vi "Main.vi"(7 "sweep rate, /min":dbl=0.2, 8 "sweep to:":dbl=4.0, 9 "sweep":T8(radio)=enum."2636a_smub") -> ()   [LabVIEW 2021] (continued)
                    n293 = property on="iTC_addr_hyper" class="VISAName"() -> ("Value"=w276:refnum<visa-resource-name>)  [unwired: 2 in, 2 out]
                    n294 = call "iTCread.vi"("VISA resource name"=w276, "iTCreadCtrl"=iTCreadCtrl."Sample Temp") -> ("number"=w277:dbl)  [unwired: 5 in, 3 out]
                  }
                }
                n295 = property on="Hyper Channel" class="DigNum (strict)"("Value"=w243) -> ()  [unwired: 2 in, 2 out]
              }
            }
          }
          frame #3 {
            # "Update current value of measured channel"
            n296 = property on="Monitor" class="Bool (strict)"() -> ("Value"=w279:bool)  [unwired: 2 in, 2 out]
            n297 = case shown="True" w279 {
              frame False {
              }
              frame True {
                n298 = stacked-sequence {
                  frame #0 {
                    # "Prepare the display format"
                    n299 = local read "2636A smua meas v"() -> (w285:bool)
                    n300 = local read "2636A smub meas v"() -> (w283:bool)
                    n301 = local read "2636A smub meas i"() -> (w282:bool)
                    n302 = local read "2636A smua meas i"() -> (w284:bool)
                    n303 = property on="sweep" class="RadioBtnsControl (strict)"() -> ("Value"=w280:T8)  [unwired: 2 in, 2 out]
                    n304 = Compound Arithmetic op=OR(w285, w284, w283, w282) -> (w281:bool)
                    n305 = case shown="True" w281 {
                      frame False {
                      }
                      frame True {
                        # "opens session for 2636a system sourcemeter"
                        n306 = local read "2614A addr"() -> (w340:refnum<visa-resource-name>)
                        n307 = VISA Close(VISA resource name=w340) -> ()  [unwired: 1 in, 1 out]
                      }
                    }
                    n308 = case shown="\"AuxOut0\"" w280 {
                      frame "2400_1" {
                        # "add label for the first column in the datafile"
                        n309 = stacked-sequence {
                          frame #0 {
                            n310 = property on="data_caption" class="Str"("Value"="") -> ()  [unwired: 2 in, 2 out]
                            n311 = property on="Figure_axis" class="Arr (strict)"("Value"=string[] [] ("Figure_axis_string")) -> ()  [unwired: 2 in, 2 out]
                          }
                          frame #1 {
                            w288 = "V_sweep_2400_1" ("V_sweep")
                            n312 = Concatenate Strings(w288, "\t") -> (w290:string)
                            n313 = Build Array(w288) -> (w289:string[])
                            n314 = property on="data_caption" class="Str"("Value"=w290) -> ()  [unwired: 2 in, 2 out]
                            n315 = property on="Figure_axis" class="Arr (strict)"("Value"=w289) -> ()  [unwired: 2 in, 2 out]
                          }
                        }
                      }
                      frame "2400_2" {
                        n316 = stacked-sequence {
                          frame #0 {
                            n317 = property on="data_caption" class="Str"("Value"="") -> ()  [unwired: 2 in, 2 out]
                            n318 = property on="Figure_axis" class="Arr (strict)"("Value"=string[] [] ("Figure_axis_string")) -> ()  [unwired: 2 in, 2 out]
                          }
                          frame #1 {
                            w294 = "V_sweep_2400_2" ("V_sweep")
                            n319 = Build Array(w294) -> (w295:string[])
                            n320 = Concatenate Strings(w294, "\t") -> (w297:string)
                            n321 = property on="Figure_axis" class="Arr (strict)"("Value"=w295) -> ()  [unwired: 2 in, 2 out]
                            n322 = property on="data_caption" class="Str"("Value"=w297) -> ()  [unwired: 2 in, 2 out]
                          }
                        }
                      }
                      frame "2400_3" {
                        n323 = stacked-sequence {
                          frame #0 {
                            n324 = property on="data_caption" class="Str"("Value"="") -> ()  [unwired: 2 in, 2 out]
                            n325 = property on="Figure_axis" class="Arr (strict)"("Value"=string[] [] ("Figure_axis_string")) -> ()  [unwired: 2 in, 2 out]
                          }
                          frame #1 {
                            w300 = "V_sweep_2400_3" ("V_sweep")
                            n326 = Concatenate Strings(w300, "\t") -> (w303:string)
                            n327 = Build Array(w300) -> (w301:string[])
                            n328 = property on="data_caption" class="Str"("Value"=w303) -> ()  [unwired: 2 in, 2 out]
                            n329 = property on="Figure_axis" class="Arr (strict)"("Value"=w301) -> ()  [unwired: 2 in, 2 out]
                          }
                        }
                      }
                      frame "2636a_smua" {
                        n330 = stacked-sequence {
                          frame #0 {
                            n331 = property on="data_caption" class="Str"("Value"="") -> ()  [unwired: 2 in, 2 out]
                            n332 = property on="Figure_axis" class="Arr (strict)"("Value"=string[] [] ("Figure_axis_string")) -> ()  [unwired: 2 in, 2 out]
                          }
                          frame #1 {
                            w306 = "V_sweep_2636a_smua" ("V_sweep")
                            n333 = Concatenate Strings(w306, "\t") -> (w309:string)
                            n334 = Build Array(w306) -> (w307:string[])
                            n335 = property on="data_caption" class="Str"("Value"=w309) -> ()  [unwired: 2 in, 2 out]
                            n336 = property on="Figure_axis" class="Arr (strict)"("Value"=w307) -> ()  [unwired: 2 in, 2 out]
                          }
                        }
                      }
                      frame "2636a_smub" {
                        n337 = stacked-sequence {
                          frame #0 {
                            n338 = property on="data_caption" class="Str"("Value"="") -> ()  [unwired: 2 in, 2 out]
                            n339 = property on="Figure_axis" class="Arr (strict)"("Value"=string[] [] ("Figure_axis_string")) -> ()  [unwired: 2 in, 2 out]
                          }
                          frame #1 {
                            w312 = "V_sweep_2636a_smub" ("V_sweep")
                            n340 = Build Array(w312) -> (w313:string[])
                            n341 = Concatenate Strings(w312, "\t") -> (w315:string)
                            n342 = property on="Figure_axis" class="Arr (strict)"("Value"=w313) -> ()  [unwired: 2 in, 2 out]
                            n343 = property on="data_caption" class="Str"("Value"=w315) -> ()  [unwired: 2 in, 2 out]
                          }
                        }
                      }
                      frame "time_sweep", Default {
                        n344 = stacked-sequence {
                          frame #0 {
                            n345 = property on="data_caption" class="Str"("Value"="") -> ()  [unwired: 2 in, 2 out]
                            n346 = property on="Figure_axis" class="Arr (strict)"("Value"=string[] [] ("Figure_axis_string")) -> ()  [unwired: 2 in, 2 out]
                          }
                          frame #1 {
                            w318 = "time_sweep" ("V_sweep")
                            n347 = Build Array(w318) -> (w319:string[])
                            n348 = Concatenate Strings(w318, "\t") -> (w320:string)
                            n349 = property on="Figure_axis" class="Arr (strict)"("Value"=w319) -> ()  [unwired: 2 in, 2 out]
                            n350 = property on="data_caption" class="Str"("Value"=w320) -> ()  [unwired: 2 in, 2 out]
                          }
                        }
                      }
                      frame "iPS" {
                        # "sweep iPS"
                        n351 = stacked-sequence {
                          frame #0 {
                            n352 = property on="data_caption" class="Str"("Value"="") -> ()  [unwired: 2 in, 2 out]
                            n353 = property on="Figure_axis" class="Arr (strict)"("Value"=string[] [] ("Figure_axis_string")) -> ()  [unwired: 2 in, 2 out]
                          }
                          frame #1 {
                            w324 = "iPS_OutputField" ("V_sweep")
                            n354 = Build Array(w324) -> (w325:string[])
                            n355 = Concatenate Strings(w324, "\t") -> (w327:string)
                            n356 = property on="Figure_axis" class="Arr (strict)"("Value"=w325) -> ()  [unwired: 2 in, 2 out]
                            n357 = property on="data_caption" class="Str"("Value"=w327) -> ()  [unwired: 2 in, 2 out]
                          }
                        }
                      }
                      frame "iTC" {
                        n358 = stacked-sequence {
                          frame #0 {
                            n359 = property on="data_caption" class="Str"("Value"="") -> ()  [unwired: 2 in, 2 out]
                            n360 = property on="Figure_axis" class="Arr (strict)"("Value"=string[] ["", "SR830_1_ip", "SR830_1_oop", "SR830_2_ip", "SR830_2_oop", "2461_meas_v", "2461_meas_i", "2636A_smua_v", "2636A_smua_i", "formula"] ("Figure_axis")) -> ()  [unwired: 2 in, 2 out]
                          }
                          frame #1 {
                            w332 = "iTC_sample"
                            n361 = Build Array(w332) -> (w331:string[])
                            n362 = Concatenate Strings(w332, "\t") -> (w330:string)
                            n363 = property on="data_caption" class="Str"("Value"=w330) -> ()  [unwired: 2 in, 2 out]
                            n364 = property on="Figure_axis" class="Arr (strict)"("Value"=w331) -> ()  [unwired: 2 in, 2 out]
                          }
                        }
                      }
                      frame "AuxOut0" {
                        n365 = stacked-sequence {
                          frame #0 {
                            n366 = property on="data_caption" class="Str"("Value"="") -> ()  [unwired: 2 in, 2 out]
                            n367 = property on="Figure_axis" class="Arr (strict)"("Value"=string[] ["", "SR830_1_ip", "SR830_1_oop", "SR830_2_ip", "SR830_2_oop", "2461_meas_v", "2461_meas_i", "2636A_smua_v", "2636A_smua_i", "formula"] ("Figure_axis")) -> ()  [unwired: 2 in, 2 out]
                          }
                          frame #1 {
                            w338 = "V_sweep_AuxOut0"
                            n368 = Build Array(w338) -> (w337:string[])
                            n369 = Concatenate Strings(w338, "\t") -> (w336:string)
                            n370 = property on="data_caption" class="Str"("Value"=w336) -> ()  [unwired: 2 in, 2 out]
                            n371 = property on="Figure_axis" class="Arr (strict)"("Value"=w337) -> ()  [unwired: 2 in, 2 out]
                          }
                        }
                      }
                    }
                  }
                  frame #1 {
                    # "0 = SR830_1_ip\n1 = SR830_1_oop\n2 = SR830_2_ip\n3 = SR830_2_oop\n4 = SR830_3_ip\n5 = SR830_3_oop\n6 = SR830_4_ip \n7 = SR830_4_oop \n8= 2400_1_v \n9 = 2400_1_i \n10 = 2400_2_v\n11 = 2400_2_i \n12 = 2400_3_v \n13 = 2400_3_i \n14 = 2182A_1_ch1 \n15 = 2182A_1_ch2 \n16 = 2182A_2_ch1 \n17 = 2182A_2_ch2\n18 = 2182A_3_ch1 \n19 = 2182A_3_ch2 \n20 = 2182A_4_ch1 \n21 = 2182A_4_ch2 \n22 = 2636A_smua_v \n23 = 2636A_smua_i \n24 = 2636A_smub_v \n25 = 2636A_smub_i \n26 = time\n27 = iPS_Field\n28 = iPS_Magnet_T\n29 = iPS__SH_T\n30 = iTC _sample_T\n31 = iTC _VTI_T\n32 = iTC _PT1_T\n33 = iTC _PT2_T\n34 = iTC _VTI_P"
                    # "this part constructs the first (text) line for the data file with names of all measured variables,\nalso constructs a text array contaning names of all measured variable for the \"ring\" (so parameter can be selected and plotted)"
                    n372 = stacked-sequence {
                      frame #0 {
                        # "SR830 1 in phase (SR830_1_ip)"
                        n373 = local read "SR830 1 ip"() -> (w345:bool)
                        n374 = property on="Figure_axis" class="Arr (strict)"() -> ("Value"=w342:string[])  [unwired: 2 in, 2 out]
                        n375 = property on="data_caption" class="Str"() -> ("Value"=w344:string)  [unwired: 2 in, 2 out]
                        n376 = case shown="True" w345 {
                          tunnel: w344 -> [w347 w353]
                          tunnel: [w347 w352] -> w343
                          tunnel: w342 -> [w346 w350]
                          tunnel: [w346 w348] -> w341
                          frame False {
                            # "not measure SR830 1 in phase signal (SR830_1_ip)"
                          }
                          frame True {
                            w349 = "SR830_1_ip"
                            # "measure SR830 1 in phase signal (SR830_1_ip)"
                            n377 = local read "SR830 1 addr"() -> (w354:u8)
                            n378 = Number To Decimal String(number=w354) -> (decimal integer string=w355:string)  [unwired: 1 in]
                            n379 = GPIB Clear(3:w355) -> ()  [unwired: 1 in, 2 out]
                            n380 = Build Array (concatenate)(w350, w349) -> (w348:string[])
                            n381 = Concatenate Strings(w353, w349, "\t") -> (w352:string)
                          }
                        }
                        n382 = property on="Figure_axis" class="Arr (strict)"("Value"=w341) -> ()  [unwired: 2 in, 2 out]
                        n383 = property on="data_caption" class="Str"("Value"=w343) -> ()  [unwired: 2 in, 2 out]
                      }
                      frame #1 {
                        # "SR830 1 out of phase (SR830_1_oop)"
                        n384 = local read "SR830 1 oop"() -> (w360:bool)
                        n385 = property on="Figure_axis" class="Arr (strict)"() -> ("Value"=w357:string[])  [unwired: 2 in, 2 out]
                        n386 = property on="data_caption" class="Str"() -> ("Value"=w359:string)  [unwired: 2 in, 2 out]
                        n387 = case shown="False" w360 {
                          tunnel: w359 -> [w362 w368]
                          tunnel: [w362 w367] -> w358
                          tunnel: w357 -> [w361 w365]
                          tunnel: [w361 w363] -> w356
                          frame False {
                            # "not measure SR830 1 out of phase signal (SR830_1_oop)"
                          }
                          frame True {
                            w364 = "SR830_1_oop"
                            # "measure SR830 1 out of phase signal (SR830_1_oop)"
                            n388 = local read "SR830 1 addr"() -> (w369:u8)
                            n389 = Number To Decimal String(number=w369) -> (decimal integer string=w370:string)  [unwired: 1 in]
                            n390 = GPIB Clear(3:w370) -> ()  [unwired: 1 in, 2 out]
                            n391 = Build Array (concatenate)(w365, w364) -> (w363:string[])
                            n392 = Concatenate Strings(w368, w364, "\t") -> (w367:string)
                          }
                        }
                        n393 = property on="Figure_axis" class="Arr (strict)"("Value"=w356) -> ()  [unwired: 2 in, 2 out]
                        n394 = property on="data_caption" class="Str"("Value"=w358) -> ()  [unwired: 2 in, 2 out]
                      }
                      frame #2 {
                        # "SR830 2 in phase (SR830_2_ip)"
                        n395 = local read "SR830 2 ip"() -> (w375:bool)
                        n396 = property on="Figure_axis" class="Arr (strict)"() -> ("Value"=w372:string[])  [unwired: 2 in, 2 out]
                        n397 = property on="data_caption" class="Str"() -> ("Value"=w374:string)  [unwired: 2 in, 2 out]
                        n398 = case shown="True" w375 {
                          tunnel: w374 -> [w377 w383]
                          tunnel: [w377 w382] -> w373
                          tunnel: w372 -> [w376 w380]
                          tunnel: [w376 w378] -> w371
                          frame False {
                            # "not measure SR830 2 in phase signal (SR830_2_ip)"
                          }
                          frame True {
                            w379 = "SR830_2_ip"
                            # "measure SR830 2 in phase signal (SR830_2_ip)"
                            n399 = local read "SR830 2 addr"() -> (w384:u8)
                            n400 = Number To Decimal String(number=w384) -> (decimal integer string=w385:string)  [unwired: 1 in]
                            n401 = GPIB Clear(3:w385) -> ()  [unwired: 1 in, 2 out]
                            n402 = Build Array (concatenate)(w380, w379) -> (w378:string[])
                            n403 = Concatenate Strings(w383, w379, "\t") -> (w382:string)
                          }
                        }
                        n404 = property on="Figure_axis" class="Arr (strict)"("Value"=w371) -> ()  [unwired: 2 in, 2 out]
                        n405 = property on="data_caption" class="Str"("Value"=w373) -> ()  [unwired: 2 in, 2 out]
                      }
                      frame #3 {
                        # "SR830 2 out of phase (SR830_2_oop)"
                        n406 = local read "SR830 2 oop"() -> (w390:bool)
                        n407 = property on="Figure_axis" class="Arr (strict)"() -> ("Value"=w387:string[])  [unwired: 2 in, 2 out]
                        n408 = property on="data_caption" class="Str"() -> ("Value"=w389:string)  [unwired: 2 in, 2 out]
                        n409 = case shown="True" w390 {
                          tunnel: w389 -> [w392 w398]
                          tunnel: [w392 w397] -> w388
                          tunnel: w387 -> [w391 w395]
                          tunnel: [w391 w393] -> w386
                          frame False {
                            # "not measure SR830 2 out of phase signal (SR830_2_oop)"
                          }
                          frame True {
                            w394 = "SR830_2_oop"
                            # "measure SR830 2 out of phase signal (SR830_2_oop)"
                            n410 = local read "SR830 2 addr"() -> (w399:u8)
                            n411 = Number To Decimal String(number=w399) -> (decimal integer string=w400:string)  [unwired: 1 in]
                            n412 = GPIB Clear(3:w400) -> ()  [unwired: 1 in, 2 out]
                            n413 = Build Array (concatenate)(w395, w394) -> (w393:string[])
                            n414 = Concatenate Strings(w398, w394, "\t") -> (w397:string)
                          }
                        }
                        n415 = property on="Figure_axis" class="Arr (strict)"("Value"=w386) -> ()  [unwired: 2 in, 2 out]
                        n416 = property on="data_caption" class="Str"("Value"=w388) -> ()  [unwired: 2 in, 2 out]
                      }
                      frame #4 {
                        # "SR830 3 in phase (SR830_3_ip)"
                        n417 = local read "SR830 3 ip"() -> (w405:bool)
                        n418 = property on="Figure_axis" class="Arr (strict)"() -> ("Value"=w402:string[])  [unwired: 2 in, 2 out]
                        n419 = property on="data_caption" class="Str"() -> ("Value"=w404:string)  [unwired: 2 in, 2 out]
                        n420 = case shown="True" w405 {
                          tunnel: w404 -> [w407 w413]
                          tunnel: [w407 w412] -> w403
                          tunnel: w402 -> [w406 w410]
                          tunnel: [w406 w408] -> w401
                          frame False {
                            # "not measure SR830 3 in phase signal (SR830_3_ip)"
                          }
                          frame True {
                            w409 = "SR830_3_ip"
                            # "measure SR830 3 in phase signal (SR830_3_ip)"
                            n421 = local read "SR830 3 addr"() -> (w414:u8)
                            n422 = Number To Decimal String(number=w414) -> (decimal integer string=w415:string)  [unwired: 1 in]
                            n423 = GPIB Clear(3:w415) -> ()  [unwired: 1 in, 2 out]
                            n424 = Build Array (concatenate)(w410, w409) -> (w408:string[])
                            n425 = Concatenate Strings(w413, w409, "\t") -> (w412:string)
                          }
                        }
                        n426 = property on="Figure_axis" class="Arr (strict)"("Value"=w401) -> ()  [unwired: 2 in, 2 out]
                        n427 = property on="data_caption" class="Str"("Value"=w403) -> ()  [unwired: 2 in, 2 out]
                      }
                      frame #5 {
                        # "SR830 3 out of phase (SR830_3_oop)"
                        n428 = local read "SR830 3 oop"() -> (w420:bool)
                        n429 = property on="Figure_axis" class="Arr (strict)"() -> ("Value"=w417:string[])  [unwired: 2 in, 2 out]
                        n430 = property on="data_caption" class="Str"() -> ("Value"=w419:string)  [unwired: 2 in, 2 out]
                        n431 = case shown="True" w420 {
                          tunnel: w419 -> [w422 w428]
                          tunnel: [w422 w427] -> w418
                          tunnel: w417 -> [w421 w425]
                          tunnel: [w421 w423] -> w416
                          frame False {
                            # "not measure SR830 3 out of phase signal (SR830_3_oop)"
                          }
                          frame True {
                            w424 = "SR830_3_oop"
                            # "measure SR830 3 out phase signal (SR830_3_oop)"
                            n432 = local read "SR830 3 addr"() -> (w429:u8)
                            n433 = Number To Decimal String(number=w429) -> (decimal integer string=w430:string)  [unwired: 1 in]
                            n434 = GPIB Clear(3:w430) -> ()  [unwired: 1 in, 2 out]
                            n435 = Build Array (concatenate)(w425, w424) -> (w423:string[])
                            n436 = Concatenate Strings(w428, w424, "\t") -> (w427:string)
                          }
                        }
                        n437 = property on="Figure_axis" class="Arr (strict)"("Value"=w416) -> ()  [unwired: 2 in, 2 out]
                        n438 = property on="data_caption" class="Str"("Value"=w418) -> ()  [unwired: 2 in, 2 out]
                      }
                      frame #6 {
                        # "SR830 4 in phase (SR830_4_ip)"
                        n439 = local read "SR830 4 ip"() -> (w435:bool)
                        n440 = property on="Figure_axis" class="Arr (strict)"() -> ("Value"=w432:string[])  [unwired: 2 in, 2 out]
                        n441 = property on="data_caption" class="Str"() -> ("Value"=w434:string)  [unwired: 2 in, 2 out]
                        n442 = case shown="True" w435 {
                          tunnel: w434 -> [w437 w443]
                          tunnel: [w437 w442] -> w433
                          tunnel: w432 -> [w436 w440]
                          tunnel: [w436 w438] -> w431
                          frame False {
                            # "not measure SR830 4 in phase signal (SR830_4_ip)"
                          }
                          frame True {
                            w439 = "SR830_4_ip"
                            # "measure SR830 4 in phase signal (SR830_4_ip)"
                            n443 = local read "SR830 4 addr"() -> (w444:u8)
                            n444 = Number To Decimal String(number=w444) -> (decimal integer string=w445:string)  [unwired: 1 in]
                            n445 = GPIB Clear(3:w445) -> ()  [unwired: 1 in, 2 out]
                            n446 = Build Array (concatenate)(w440, w439) -> (w438:string[])
                            n447 = Concatenate Strings(w443, w439, "\t") -> (w442:string)
                          }
                        }
                        n448 = property on="Figure_axis" class="Arr (strict)"("Value"=w431) -> ()  [unwired: 2 in, 2 out]
                        n449 = property on="data_caption" class="Str"("Value"=w433) -> ()  [unwired: 2 in, 2 out]
                      }
                      frame #7 {
                        # "SR830 4 out of phase (SR830_4_oop)"
                        n450 = local read "SR830 4 oop"() -> (w450:bool)
                        n451 = property on="Figure_axis" class="Arr (strict)"() -> ("Value"=w447:string[])  [unwired: 2 in, 2 out]
                        n452 = property on="data_caption" class="Str"() -> ("Value"=w449:string)  [unwired: 2 in, 2 out]
                        n453 = case shown="True" w450 {
                          tunnel: w449 -> [w452 w458]
                          tunnel: [w452 w457] -> w448
                          tunnel: w447 -> [w451 w455]
                          tunnel: [w451 w453] -> w446
                          frame False {
                            # "not measure SR830 4 out of phase signal (SR830_4_oop)"
                          }
                          frame True {
                            w454 = "SR830_4_oop"
                            # "measure SR830 4 out of phase signal (SR830_4_oop)"
                            n454 = local read "SR830 4 addr"() -> (w459:u8)
                            n455 = Number To Decimal String(number=w459) -> (decimal integer string=w460:string)  [unwired: 1 in]
                            n456 = GPIB Clear(3:w460) -> ()  [unwired: 1 in, 2 out]
                            n457 = Build Array (concatenate)(w455, w454) -> (w453:string[])
                            n458 = Concatenate Strings(w458, w454, "\t") -> (w457:string)
                          }
                        }
                        n459 = property on="Figure_axis" class="Arr (strict)"("Value"=w446) -> ()  [unwired: 2 in, 2 out]
                        n460 = property on="data_caption" class="Str"("Value"=w448) -> ()  [unwired: 2 in, 2 out]
                      }
                      frame #8 {
                        # "2400 1 voltage measure (2400_1_v)"
                        n461 = local read "2400 1 meas v"() -> (w465:bool)
                        n462 = property on="Figure_axis" class="Arr (strict)"() -> ("Value"=w462:string[])  [unwired: 2 in, 2 out]
                        n463 = property on="data_caption" class="Str"() -> ("Value"=w464:string)  [unwired: 2 in, 2 out]
                        n464 = case shown="True" w465 {
                          tunnel: w464 -> [w467 w473]
                          tunnel: [w467 w472] -> w463
                          tunnel: w462 -> [w466 w470]
                          tunnel: [w466 w468] -> w461
                          frame False {
                            # "not measure 2400 1 voltage (2400_1_v)"
                          }
                          frame True {
                            w469 = "2400_1_v"
                            # "measure 2400 1 voltage (2400_1_v)"
                            n465 = local read "2400 1 addr"() -> (w474:u8)
                            n466 = Number To Decimal String(number=w474) -> (decimal integer string=w475:string)  [unwired: 1 in]
                            n467 = GPIB Clear(3:w475) -> ()  [unwired: 1 in, 2 out]
                            n468 = Build Array (concatenate)(w470, w469) -> (w468:string[])
                            n469 = Concatenate Strings(w473, w469, "\t") -> (w472:string)
                          }
                        }
                        n470 = property on="Figure_axis" class="Arr (strict)"("Value"=w461) -> ()  [unwired: 2 in, 2 out]
                        n471 = property on="data_caption" class="Str"("Value"=w463) -> ()  [unwired: 2 in, 2 out]
                      }
                      frame #9 {
                        # "2400 1 current measure (2400_1_i)"
                        n472 = local read "2400 1 meas i"() -> (w480:bool)
                        n473 = property on="Figure_axis" class="Arr (strict)"() -> ("Value"=w477:string[])  [unwired: 2 in, 2 out]
                        n474 = property on="data_caption" class="Str"() -> ("Value"=w479:string)  [unwired: 2 in, 2 out]
                        n475 = case shown="True" w480 {
                          tunnel: w479 -> [w482 w488]
                          tunnel: [w482 w487] -> w478
                          tunnel: w477 -> [w481 w485]
                          tunnel: [w481 w483] -> w476
                          frame False {
                            # "not measure 2400 1 current (2400_1_i)"
                          }
                          frame True {
                            w484 = "2400_1_i"
                            # "measure 2400 1 current (2400_1_i)"
                            n476 = local read "2400 1 addr"() -> (w489:u8)
                            n477 = Number To Decimal String(number=w489) -> (decimal integer string=w490:string)  [unwired: 1 in]
                            n478 = GPIB Clear(3:w490) -> ()  [unwired: 1 in, 2 out]
                            n479 = Build Array (concatenate)(w485, w484) -> (w483:string[])
                            n480 = Concatenate Strings(w488, w484, "\t") -> (w487:string)
                          }
                        }
                        n481 = property on="Figure_axis" class="Arr (strict)"("Value"=w476) -> ()  [unwired: 2 in, 2 out]
                        n482 = property on="data_caption" class="Str"("Value"=w478) -> ()  [unwired: 2 in, 2 out]
                      }
                      frame #10 {
                        # "2400 2 voltage measure (2400_2_v)"
                        n483 = local read "2400 2 meas v"() -> (w495:bool)
                        n484 = property on="Figure_axis" class="Arr (strict)"() -> ("Value"=w492:string[])  [unwired: 2 in, 2 out]
                        n485 = property on="data_caption" class="Str"() -> ("Value"=w494:string)  [unwired: 2 in, 2 out]
                        n486 = case shown="True" w495 {
                          tunnel: w494 -> [w497 w503]
                          tunnel: [w497 w502] -> w493
                          tunnel: w492 -> [w496 w500]
                          tunnel: [w496 w498] -> w491
                          frame False {
                            # "not measure 2400 2 voltage (2400_2_v)"
                          }
                          frame True {
                            w499 = "2400_2_v"
                            # "measure 2400 2 voltage (2400_2_v)"
                            n487 = local read "2400 2 addr"() -> (w504:u8)
                            n488 = Number To Decimal String(number=w504) -> (decimal integer string=w505:string)  [unwired: 1 in]
                            n489 = GPIB Clear(3:w505) -> ()  [unwired: 1 in, 2 out]
                            n490 = Build Array (concatenate)(w500, w499) -> (w498:string[])
                            n491 = Concatenate Strings(w503, w499, "\t") -> (w502:string)
                          }
                        }
                        n492 = property on="Figure_axis" class="Arr (strict)"("Value"=w491) -> ()  [unwired: 2 in, 2 out]
                        n493 = property on="data_caption" class="Str"("Value"=w493) -> ()  [unwired: 2 in, 2 out]
                      }
                      frame #11 {
                        # "2400 2 current measure (2400_2_i)"
                        n494 = local read "2400 2 meas i"() -> (w510:bool)
                        n495 = property on="Figure_axis" class="Arr (strict)"() -> ("Value"=w507:string[])  [unwired: 2 in, 2 out]
                        n496 = property on="data_caption" class="Str"() -> ("Value"=w509:string)  [unwired: 2 in, 2 out]
                        n497 = case shown="True" w510 {
                          tunnel: w509 -> [w512 w518]
                          tunnel: [w512 w517] -> w508
                          tunnel: w507 -> [w511 w515]
                          tunnel: [w511 w513] -> w506
                          frame False {
                            # "not measure 2400 2 current (2400_2_i)"
                          }
                          frame True {
                            w514 = "2400_2_i"
                            # "measure 2400 2 current (2400_2_i)"
                            n498 = local read "2400 2 addr"() -> (w519:u8)
                            n499 = Number To Decimal String(number=w519) -> (decimal integer string=w520:string)  [unwired: 1 in]
                            n500 = GPIB Clear(3:w520) -> ()  [unwired: 1 in, 2 out]
                            n501 = Build Array (concatenate)(w515, w514) -> (w513:string[])
                            n502 = Concatenate Strings(w518, w514, "\t") -> (w517:string)
                          }
                        }
                        n503 = property on="Figure_axis" class="Arr (strict)"("Value"=w506) -> ()  [unwired: 2 in, 2 out]
                        n504 = property on="data_caption" class="Str"("Value"=w508) -> ()  [unwired: 2 in, 2 out]
                      }
                      frame #12 {
                        # "2400 3 voltage measure (2400_3_v)"
                        n505 = local read "2400 3 meas v"() -> (w525:bool)
                        n506 = property on="Figure_axis" class="Arr (strict)"() -> ("Value"=w522:string[])  [unwired: 2 in, 2 out]
                        n507 = property on="data_caption" class="Str"() -> ("Value"=w524:string)  [unwired: 2 in, 2 out]
                        n508 = case shown="True" w525 {
                          tunnel: w524 -> [w527 w533]
                          tunnel: [w527 w532] -> w523
                          tunnel: w522 -> [w526 w530]
                          tunnel: [w526 w528] -> w521
                          frame False {
                            # "not measure 2400 3 voltage (2400_3_v)"
                          }
                          frame True {
                            w529 = "2400_3_v"
                            # "measure 2400 3 voltage (2400_3_v)"
                            n509 = local read "2400 3 addr"() -> (w534:u8)
                            n510 = Number To Decimal String(number=w534) -> (decimal integer string=w535:string)  [unwired: 1 in]
                            n511 = GPIB Clear(3:w535) -> ()  [unwired: 1 in, 2 out]
                            n512 = Build Array (concatenate)(w530, w529) -> (w528:string[])
                            n513 = Concatenate Strings(w533, w529, "\t") -> (w532:string)
                          }
                        }
                        n514 = property on="Figure_axis" class="Arr (strict)"("Value"=w521) -> ()  [unwired: 2 in, 2 out]
                        n515 = property on="data_caption" class="Str"("Value"=w523) -> ()  [unwired: 2 in, 2 out]
                      }
                      frame #13 {
                        # "2400 3 current measure (2400_3_i)"
                        n516 = local read "2400 3 meas i"() -> (w540:bool)
                        n517 = property on="Figure_axis" class="Arr (strict)"() -> ("Value"=w537:string[])  [unwired: 2 in, 2 out]
                        n518 = property on="data_caption" class="Str"() -> ("Value"=w539:string)  [unwired: 2 in, 2 out]
                        n519 = case shown="True" w540 {
                          tunnel: w539 -> [w542 w548]
                          tunnel: [w542 w547] -> w538
                          tunnel: w537 -> [w541 w545]
                          tunnel: [w541 w543] -> w536
                          frame False {
                            # "not measure 2400 3 current (2400_3_i)"
                          }
                          frame True {
                            w544 = "2400_3_i"
                            # "measure 2400 3 current (2400_3_i)"
                            n520 = local read "2400 3 addr"() -> (w549:u8)
                            n521 = Number To Decimal String(number=w549) -> (decimal integer string=w550:string)  [unwired: 1 in]
                            n522 = GPIB Clear(3:w550) -> ()  [unwired: 1 in, 2 out]
                            n523 = Build Array (concatenate)(w545, w544) -> (w543:string[])
                            n524 = Concatenate Strings(w548, w544, "\t") -> (w547:string)
                          }
                        }
                        n525 = property on="Figure_axis" class="Arr (strict)"("Value"=w536) -> ()  [unwired: 2 in, 2 out]
                        n526 = property on="data_caption" class="Str"("Value"=w538) -> ()  [unwired: 2 in, 2 out]
                      }
                      frame #14 {
                        # "2182A 1 channel 1 measure (2182A_1_ch1)"
                        n527 = local read "2182A 1 ch1"() -> (w555:bool)
                        n528 = property on="Figure_axis" class="Arr (strict)"() -> ("Value"=w552:string[])  [unwired: 2 in, 2 out]
                        n529 = property on="data_caption" class="Str"() -> ("Value"=w554:string)  [unwired: 2 in, 2 out]
                        n530 = case shown="False" w555 {
                          tunnel: w554 -> [w557 w563]
                          tunnel: [w557 w562] -> w553
                          tunnel: w552 -> [w556 w560]
                          tunnel: [w556 w558] -> w551
                          frame False {
                            # "not measure 2182A 1 channel 1 (2182A_1_ch1)"
                          }
                          frame True {
                            w559 = "2182A_1_ch1"
                            # "measure 2182A 1 channel 1 (2182A_1_ch1)"
                            n531 = local read "2182A 1 addr"() -> (w564:u8)
                            n532 = Number To Decimal String(number=w564) -> (decimal integer string=w565:string)  [unwired: 1 in]
                            n533 = GPIB Clear(3:w565) -> ()  [unwired: 1 in, 2 out]
                            n534 = Build Array (concatenate)(w560, w559) -> (w558:string[])
                            n535 = Concatenate Strings(w563, w559, "\t") -> (w562:string)
                          }
                        }
                        n536 = property on="Figure_axis" class="Arr (strict)"("Value"=w551) -> ()  [unwired: 2 in, 2 out]
                        n537 = property on="data_caption" class="Str"("Value"=w553) -> ()  [unwired: 2 in, 2 out]
                      }
                      frame #15 {
                        # "2182A 1 channel 2 measure (2182A_1_ch2)"
                        n538 = local read "2182A 1 ch2"() -> (w570:bool)
                        n539 = property on="Figure_axis" class="Arr (strict)"() -> ("Value"=w567:string[])  [unwired: 2 in, 2 out]
                        n540 = property on="data_caption" class="Str"() -> ("Value"=w569:string)  [unwired: 2 in, 2 out]
                        n541 = case shown="True" w570 {
                          tunnel: w569 -> [w572 w578]
                          tunnel: [w572 w577] -> w568
                          tunnel: w567 -> [w571 w575]
                          tunnel: [w571 w573] -> w566
                          frame False {
                            # "not measure 2182A 1 channel 2 (2182A_1_ch2)"
                          }
                          frame True {
                            w574 = "2182A_1_ch2"
                            # "measure 2182A 1 channel 2 (2182A_1_ch2)"
                            n542 = local read "2182A 1 addr"() -> (w579:u8)
                            n543 = Number To Decimal String(number=w579) -> (decimal integer string=w580:string)  [unwired: 1 in]
                            n544 = GPIB Clear(3:w580) -> ()  [unwired: 1 in, 2 out]
                            n545 = Build Array (concatenate)(w575, w574) -> (w573:string[])
                            n546 = Concatenate Strings(w578, w574, "\t") -> (w577:string)
                          }
                        }
                        n547 = property on="Figure_axis" class="Arr (strict)"("Value"=w566) -> ()  [unwired: 2 in, 2 out]
                        n548 = property on="data_caption" class="Str"("Value"=w568) -> ()  [unwired: 2 in, 2 out]
                      }
                      frame #16 {
                        # "2182A 2 channel 1 measure (2182A_2_ch1)"
                        n549 = local read "2182A 2 ch1"() -> (w585:bool)
                        n550 = property on="Figure_axis" class="Arr (strict)"() -> ("Value"=w582:string[])  [unwired: 2 in, 2 out]
                        n551 = property on="data_caption" class="Str"() -> ("Value"=w584:string)  [unwired: 2 in, 2 out]
                        n552 = case shown="True" w585 {
                          tunnel: w584 -> [w587 w593]
                          tunnel: [w587 w592] -> w583
                          tunnel: w582 -> [w586 w590]
                          tunnel: [w586 w588] -> w581
                          frame False {
                            # "not measure 2182A 2 channel 1 (2182A_2_ch1)"
                          }
                          frame True {
                            w589 = "2182A_2_ch1"
                            # "measure 2182A 2 channel 1 (2182A_2_ch1)"
                            n553 = local read "2182A 2 addr"() -> (w594:u8)
                            n554 = Number To Decimal String(number=w594) -> (decimal integer string=w595:string)  [unwired: 1 in]
                            n555 = GPIB Clear(3:w595) -> ()  [unwired: 1 in, 2 out]
                            n556 = Build Array (concatenate)(w590, w589) -> (w588:string[])
                            n557 = Concatenate Strings(w593, w589, "\t") -> (w592:string)
                          }
                        }
                        n558 = property on="Figure_axis" class="Arr (strict)"("Value"=w581) -> ()  [unwired: 2 in, 2 out]
                        n559 = property on="data_caption" class="Str"("Value"=w583) -> ()  [unwired: 2 in, 2 out]
                      }
                      frame #17 {
                        # "2182A 2 channel 2 measure (2182A_2_ch2)"
                        n560 = local read "2182A 2 ch2"() -> (w600:bool)
                        n561 = property on="Figure_axis" class="Arr (strict)"() -> ("Value"=w597:string[])  [unwired: 2 in, 2 out]
                        n562 = property on="data_caption" class="Str"() -> ("Value"=w599:string)  [unwired: 2 in, 2 out]
                        n563 = case shown="True" w600 {
                          tunnel: w599 -> [w602 w608]
                          tunnel: [w602 w607] -> w598
                          tunnel: w597 -> [w601 w605]
                          tunnel: [w601 w603] -> w596
                          frame False {
                            # "not measure 2182A 2 channel 2 (2182A_2_ch2)"
                          }
                          frame True {
                            w604 = "2182A_2_ch2"
                            # "measure 2182A 2 channel 2 (2182A_2_ch2)"
                            n564 = local read "2182A 2 addr"() -> (w609:u8)
                            n565 = Number To Decimal String(number=w609) -> (decimal integer string=w610:string)  [unwired: 1 in]
                            n566 = GPIB Clear(3:w610) -> ()  [unwired: 1 in, 2 out]
                            n567 = Build Array (concatenate)(w605, w604) -> (w603:string[])
                            n568 = Concatenate Strings(w608, w604, "\t") -> (w607:string)
                          }
                        }
                        n569 = property on="Figure_axis" class="Arr (strict)"("Value"=w596) -> ()  [unwired: 2 in, 2 out]
                        n570 = property on="data_caption" class="Str"("Value"=w598) -> ()  [unwired: 2 in, 2 out]
                      }
                      frame #18 {
                        # "2182A 3 channel 1 measure (2182A_3_ch1)"
                        n571 = local read "2182A 3 ch1"() -> (w615:bool)
                        n572 = property on="Figure_axis" class="Arr (strict)"() -> ("Value"=w612:string[])  [unwired: 2 in, 2 out]
                        n573 = property on="data_caption" class="Str"() -> ("Value"=w614:string)  [unwired: 2 in, 2 out]
                        n574 = case shown="True" w615 {
                          tunnel: w614 -> [w617 w623]
                          tunnel: [w617 w622] -> w613
                          tunnel: w612 -> [w616 w620]
                          tunnel: [w616 w618] -> w611
                          frame False {
                            # "not measure 2182A 3 channel 1 (2182A_3_ch1)"
                          }
                          frame True {
                            w619 = "2182A_3_ch1"
                            # "measure 2182A 3 channel 1 (2182A_3_ch1)"
                            n575 = local read "2182A 3 addr"() -> (w624:u8)
                            n576 = Number To Decimal String(number=w624) -> (decimal integer string=w625:string)  [unwired: 1 in]
                            n577 = GPIB Clear(3:w625) -> ()  [unwired: 1 in, 2 out]
                            n578 = Build Array (concatenate)(w620, w619) -> (w618:string[])
                            n579 = Concatenate Strings(w623, w619, "\t") -> (w622:string)
                          }
                        }
                        n580 = property on="Figure_axis" class="Arr (strict)"("Value"=w611) -> ()  [unwired: 2 in, 2 out]
                        n581 = property on="data_caption" class="Str"("Value"=w613) -> ()  [unwired: 2 in, 2 out]
                      }
                      frame #19 {
                        # "2182A 3 channel 2 measure (2182A_3_ch2)"
                        n582 = local read "2182A 3 ch2"() -> (w630:bool)
                        n583 = property on="Figure_axis" class="Arr (strict)"() -> ("Value"=w627:string[])  [unwired: 2 in, 2 out]
                        n584 = property on="data_caption" class="Str"() -> ("Value"=w629:string)  [unwired: 2 in, 2 out]
                        n585 = case shown="False" w630 {
                          tunnel: w629 -> [w632 w638]
                          tunnel: [w632 w637] -> w628
                          tunnel: w627 -> [w631 w635]
                          tunnel: [w631 w633] -> w626
                          frame False {
                            # "not measure 2182A 3 channel 2 (2182A_3_ch2)"
                          }
                          frame True {
                            w634 = "2182A_3_ch2"
                            # "measure 2182A 3 channel 2 (2182A_3_ch2)"
                            n586 = local read "2182A 3 addr"() -> (w639:u8)
                            n587 = Number To Decimal String(number=w639) -> (decimal integer string=w640:string)  [unwired: 1 in]
                            n588 = GPIB Clear(3:w640) -> ()  [unwired: 1 in, 2 out]
                            n589 = Build Array (concatenate)(w635, w634) -> (w633:string[])
                            n590 = Concatenate Strings(w638, w634, "\t") -> (w637:string)
                          }
                        }
                        n591 = property on="Figure_axis" class="Arr (strict)"("Value"=w626) -> ()  [unwired: 2 in, 2 out]
                        n592 = property on="data_caption" class="Str"("Value"=w628) -> ()  [unwired: 2 in, 2 out]
                      }
                      frame #20 {
                        # "2182A 4 channel 1 measure (2182A_4_ch1)"
                        n593 = local read "2182A 4 ch1"() -> (w645:bool)
                        n594 = property on="Figure_axis" class="Arr (strict)"() -> ("Value"=w642:string[])  [unwired: 2 in, 2 out]
                        n595 = property on="data_caption" class="Str"() -> ("Value"=w644:string)  [unwired: 2 in, 2 out]
                        n596 = case shown="True" w645 {
                          tunnel: w644 -> [w647 w653]
                          tunnel: [w647 w652] -> w643
                          tunnel: w642 -> [w646 w650]
                          tunnel: [w646 w648] -> w641
                          frame False {
                            # "not measure 2182A 4 channel 1 (2182A_4_ch1)"
                          }
                          frame True {
                            w649 = "2182A_4_ch1"
                            # "measure 2182A 4 channel 1 (2182A_4_ch1)"
                            n597 = local read "2182A 4 addr"() -> (w654:u8)
                            n598 = Number To Decimal String(number=w654) -> (decimal integer string=w655:string)  [unwired: 1 in]
                            n599 = GPIB Clear(3:w655) -> ()  [unwired: 1 in, 2 out]
                            n600 = Build Array (concatenate)(w650, w649) -> (w648:string[])
                            n601 = Concatenate Strings(w653, w649, "\t") -> (w652:string)
                          }
                        }
                        n602 = property on="Figure_axis" class="Arr (strict)"("Value"=w641) -> ()  [unwired: 2 in, 2 out]
                        n603 = property on="data_caption" class="Str"("Value"=w643) -> ()  [unwired: 2 in, 2 out]
                      }
                      frame #21 {
                        # "2182A 4 channel 2 measure (2182A_4_ch2)"
                        n604 = local read "2182A 4 ch2"() -> (w660:bool)
                        n605 = property on="Figure_axis" class="Arr (strict)"() -> ("Value"=w657:string[])  [unwired: 2 in, 2 out]
                        n606 = property on="data_caption" class="Str"() -> ("Value"=w659:string)  [unwired: 2 in, 2 out]
                        n607 = case shown="True" w660 {
                          tunnel: w659 -> [w662 w668]
                          tunnel: [w662 w667] -> w658
                          tunnel: w657 -> [w661 w665]
                          tunnel: [w661 w663] -> w656
                          frame False {
                            # "not measure 2182A 4 channel 2 (2182A_4_ch2)"
                          }
                          frame True {
                            w664 = "2182A_4_ch2"
                            # "measure 2182A 4 channel 2 (2182A_4_ch2)"
                            n608 = local read "2182A 4 addr"() -> (w669:u8)
                            n609 = Number To Decimal String(number=w669) -> (decimal integer string=w670:string)  [unwired: 1 in]
                            n610 = GPIB Clear(3:w670) -> ()  [unwired: 1 in, 2 out]
                            n611 = Build Array (concatenate)(w665, w664) -> (w663:string[])
                            n612 = Concatenate Strings(w668, w664, "\t") -> (w667:string)
                          }
                        }
                        n613 = property on="Figure_axis" class="Arr (strict)"("Value"=w656) -> ()  [unwired: 2 in, 2 out]
                        n614 = property on="data_caption" class="Str"("Value"=w658) -> ()  [unwired: 2 in, 2 out]
                      }
                      frame #22 {
                        # "2636A smua measure voltage (2636A_smua_v)"
                        n615 = local read "2636A smua meas v"() -> (w675:bool)
                        n616 = property on="Figure_axis" class="Arr (strict)"() -> ("Value"=w672:string[])  [unwired: 2 in, 2 out]
                        n617 = property on="data_caption" class="Str"() -> ("Value"=w674:string)  [unwired: 2 in, 2 out]
                        n618 = case shown="True" w675 {
                          tunnel: w674 -> [w677 w688]
                          tunnel: [w677 w687] -> w673
                          tunnel: w672 -> [w676 w685]
                          tunnel: [w676 w683] -> w671
                          frame False {
                            # "not measure voltage on 2636A smua (2636A_smua_v)"
                          }
                          frame True {
                            w684 = "2636A_smua_v"
                            # "measure voltage on 2636A smua (2636A_smua_v)"
                            n619 = local read "2614A addr"() -> (w679:refnum<visa-resource-name>)
                            n620 = VISA Open(VISA resource name=w679) -> (VISA resource name=w678:refnum<visa-resource-name>, error out=w680:errorcluster)  [unwired: 4 in]
                            n621 = VISA Clear(VISA resource name=w678, error in (no error)=w680) -> (VISA resource name out=w682:refnum<visa-resource-name>)  [unwired: 1 out]
                            n622 = property class="Instr"(reference=w682, "General Settings:Timeout Value"=u32 10000) -> ()  [unwired: 1 in, 2 out]
                            n623 = Build Array (concatenate)(w685, w684) -> (w683:string[])
                            n624 = Concatenate Strings(w688, w684, "\t") -> (w687:string)
                          }
                        }
                        n625 = property on="Figure_axis" class="Arr (strict)"("Value"=w671) -> ()  [unwired: 2 in, 2 out]
                        n626 = property on="data_caption" class="Str"("Value"=w673) -> ()  [unwired: 2 in, 2 out]
                      }
                      frame #23 {
                        # "2636A smua measure current (2636A_smua_i)"
                        n627 = local read "2636A smua meas i"() -> (w693:bool)
                        n628 = property on="Figure_axis" class="Arr (strict)"() -> ("Value"=w690:string[])  [unwired: 2 in, 2 out]
                        n629 = property on="data_caption" class="Str"() -> ("Value"=w692:string)  [unwired: 2 in, 2 out]
                        n630 = case shown="True" w693 {
                          tunnel: w692 -> [w695 w706]
                          tunnel: [w695 w705] -> w691
                          tunnel: w690 -> [w694 w703]
                          tunnel: [w694 w701] -> w689
                          frame False {
                            # "not measure current on 2636A smua (2636A_smua_i)"
                          }
                          frame True {
                            w702 = "2636A_smua_i"
                            # "measure current on 2636A smua (2636A_smua_i)"
                            n631 = local read "2614A addr"() -> (w698:refnum<visa-resource-name>)
                            n632 = VISA Open(VISA resource name=w698) -> (VISA resource name=w697:refnum<visa-resource-name>, error out=w696:errorcluster)  [unwired: 4 in]
                            n633 = VISA Clear(VISA resource name=w697, error in (no error)=w696) -> (VISA resource name out=w699:refnum<visa-resource-name>)  [unwired: 1 out]
                            n634 = Build Array (concatenate)(w703, w702) -> (w701:string[])
                            n635 = property class="Instr"(reference=w699, "General Settings:Timeout Value"=u32 10000) -> ()  [unwired: 1 in, 2 out]
                            n636 = Concatenate Strings(w706, w702, "\t") -> (w705:string)
                          }
                        }
                        n637 = property on="Figure_axis" class="Arr (strict)"("Value"=w689) -> ()  [unwired: 2 in, 2 out]
                        n638 = property on="data_caption" class="Str"("Value"=w691) -> ()  [unwired: 2 in, 2 out]
                      }
                      frame #24 {
                        # "2636A smub measure voltage (2636A_smub_v)"
                        n639 = local read "2636A smub meas v"() -> (w711:bool)
                        n640 = property on="Figure_axis" class="Arr (strict)"() -> ("Value"=w708:string[])  [unwired: 2 in, 2 out]
                        n641 = property on="data_caption" class="Str"() -> ("Value"=w710:string)  [unwired: 2 in, 2 out]
                        n642 = case shown="True" w711 {
                          tunnel: w710 -> [w713 w724]
                          tunnel: [w713 w723] -> w709
                          tunnel: w708 -> [w712 w721]
                          tunnel: [w712 w719] -> w707
                          frame False {
                            # "not measure voltage on 2636A smub (2636A_smub_v)"
                          }
                          frame True {
                            w720 = "2636A_smub_v"
                            # "measure voltage on 2636A smub (2636A_smub_v)"
                            n643 = local read "2614A addr"() -> (w715:refnum<visa-resource-name>)
                            n644 = VISA Open(VISA resource name=w715) -> (VISA resource name=w714:refnum<visa-resource-name>, error out=w716:errorcluster)  [unwired: 4 in]
                            n645 = VISA Clear(VISA resource name=w714, error in (no error)=w716) -> (VISA resource name out=w717:refnum<visa-resource-name>)  [unwired: 1 out]
                            n646 = Build Array (concatenate)(w721, w720) -> (w719:string[])
                            n647 = property class="Instr"(reference=w717, "General Settings:Timeout Value"=u32 10000) -> ()  [unwired: 1 in, 2 out]
                            n648 = Concatenate Strings(w724, w720, "\t") -> (w723:string)
                          }
                        }
                        n649 = property on="Figure_axis" class="Arr (strict)"("Value"=w707) -> ()  [unwired: 2 in, 2 out]
                        n650 = property on="data_caption" class="Str"("Value"=w709) -> ()  [unwired: 2 in, 2 out]
                      }
                      frame #25 {
                        # "2636A smub measure current (2636A_smub_i)"
                        n651 = local read "2636A smub meas i"() -> (w729:bool)
                        n652 = property on="Figure_axis" class="Arr (strict)"() -> ("Value"=w726:string[])  [unwired: 2 in, 2 out]
                        n653 = property on="data_caption" class="Str"() -> ("Value"=w728:string)  [unwired: 2 in, 2 out]
                        n654 = case shown="True" w729 {
                          tunnel: w728 -> [w731 w742]
                          tunnel: [w731 w741] -> w727
                          tunnel: w726 -> [w730 w739]
                          tunnel: [w730 w737] -> w725
                          frame False {
                            # "not measure current on 2636A smub (2636A_smub_i)"
                          }
                          frame True {
                            w738 = "2636A_smub_i"
                            # "measure current on 2636A smub (2636A_smub_i)"
                            n655 = local read "2614A addr"() -> (w732:refnum<visa-resource-name>)
                            n656 = VISA Open(VISA resource name=w732) -> (VISA resource name=w733:refnum<visa-resource-name>, error out=w734:errorcluster)  [unwired: 4 in]
                            n657 = VISA Clear(VISA resource name=w733, error in (no error)=w734) -> (VISA resource name out=w735:refnum<visa-resource-name>)  [unwired: 1 out]
                            n658 = Build Array (concatenate)(w739, w738) -> (w737:string[])
                            n659 = property class="Instr"(reference=w735, "General Settings:Timeout Value"=u32 10000) -> ()  [unwired: 1 in, 2 out]
                            n660 = Concatenate Strings(w742, w738, "\t") -> (w741:string)
                          }
                        }
                        n661 = property on="Figure_axis" class="Arr (strict)"("Value"=w725) -> ()  [unwired: 2 in, 2 out]
